vi "SQLite Upsert.vi"(4 "Where clause":string, 5 "Column/Value Pairs":string[][](array[string]), 6 "错误输入（无错误）":errorcluster, 7 "Table Name":string, 8 "Constraint Columns":string[](array[string]), 9 "DB Path":string) -> (0 "错误输出":errorcluster, 2 "Last Insert Row ID":u64, 3 "DB Path Out":string)   [LabVIEW 2016]
uses:
  <userlib>/_LVST/sqlite_api/Core/Insert/SQLite_Upsert.vi
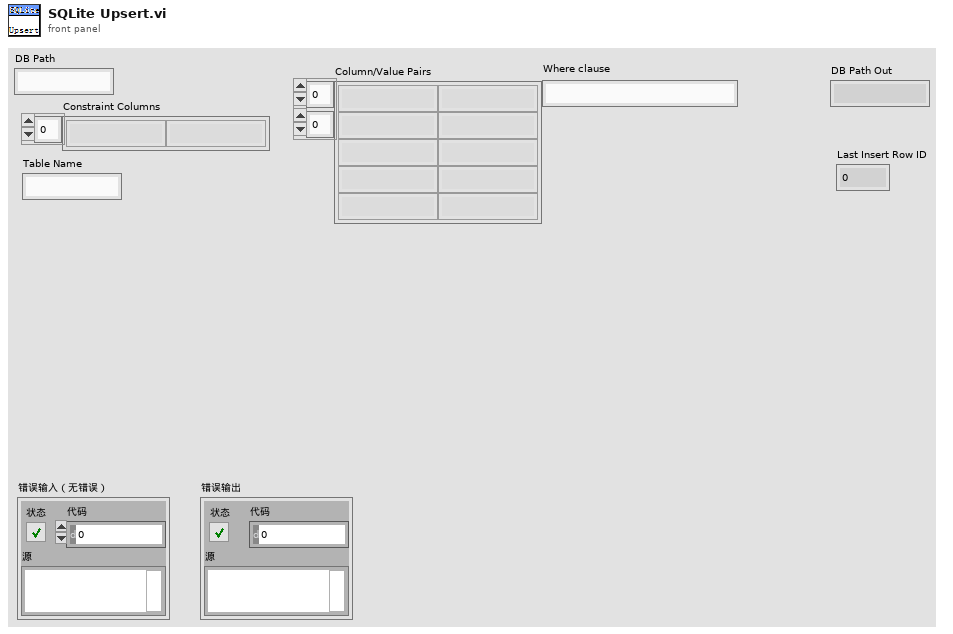
[diagram p1: front panel]
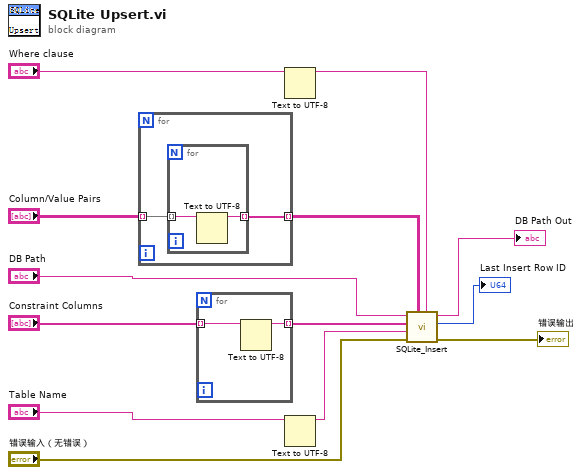
[diagram p0: block diagram]
diagram:
  n1 = for {
    tunnel: "Column/Value Pairs" -> [w15] mode=indexing
    tunnel: [w14] -> w3 mode=indexing
    n2 = for {
      tunnel: w15 -> [w17] mode=indexing
      tunnel: [w16] -> w14 mode=indexing
      n3 = Text to UTF-8(11:w17) -> (3:w16:string)  [unwired: 2 in, 1 out]
    }
  }
  n4 = for {
    tunnel: "Constraint Columns" -> [w19] mode=indexing
    tunnel: [w18] -> w1 mode=indexing
    n5 = Text to UTF-8(11:w19) -> (3:w18:string)  [unwired: 2 in, 1 out]
  }
  n6 = Text to UTF-8(11:"Where clause") -> (3:w5:string)  [unwired: 2 in, 1 out]
  n7 = Text to UTF-8(11:"Table Name") -> (3:w7:string)  [unwired: 2 in, 1 out]
  n8 = call-poly <userlib>:"SQLite_Insert.vi"("Where clause"=w5, "Column/Value Pairs"=w3, "error in"="错误输入（无错误）", "Table Name"=w7, "Constraint Columns"=w1, "DB Path"="DB Path") -> ("error out"=→"错误输出":errorcluster, "Last Insert Row ID"=→"Last Insert Row ID":u64, "DB Path Out"=→"DB Path Out":string)  [unwired: 1 in]
